vi "writeToXML.vi"(8 "error in (no error)":errorcluster, 10 "Class Label":string="GuideTargetPosition", 11 "GuideTargetPosition in":refnum<class "GuideTargetPosition.lvclass">) -> (0 "error out":errorcluster, 2 "outputXMLString":string="<GuideTargetPosition>\n  <target>\n    <gTargTime>0</gTargTime>\n    <trackID>0</trackID>\n    <xPosition_mm>0</xPosition_mm>\n    <yPosition_mm>0</yPosition_mm>\n  </target>\n</GuideTargetPosition>", 3 "GuideTargetPosition out":refnum<class "GuideTargetPosition.lvclass">)   [LabVIEW 2022 SP3, in "TCSDataDefinitions.lvlib" / "TCSGuiderStatus.lvlib" / "GuideTargetPosition.lvclass"]
uses:
  GuideTargetPosition.lvclass
  GuideTargetPosition.lvclass/GuideTargetPosition.ctl
  TCSGuiderStatus/TCSGuideStatus.lvclass
  GWTargetPositionParameters/GWTargetPositionParameters.lvclass
  <userlib>/Common/XML/XMLGenerator/XMLGenerator.lvclass
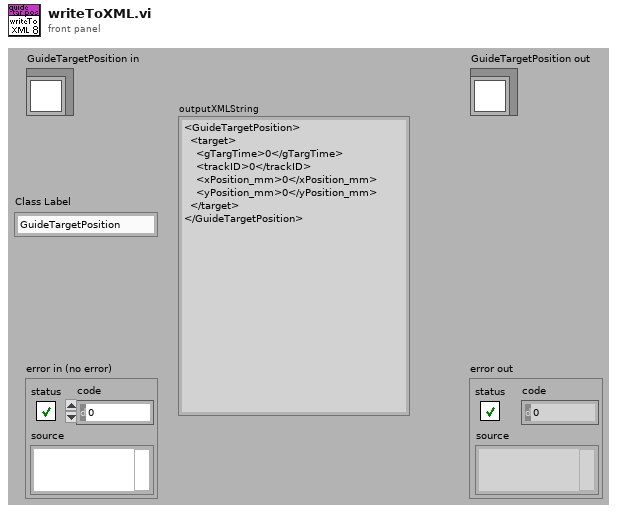
[diagram p1: front panel]
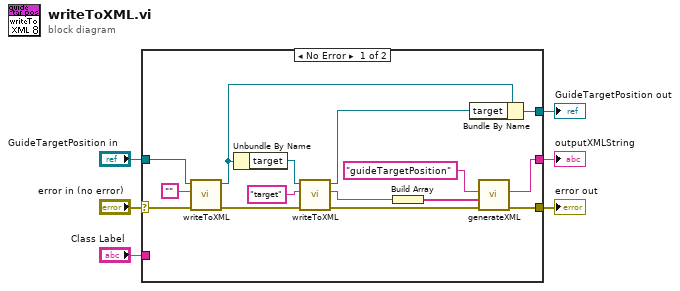
[diagram p0: block diagram]
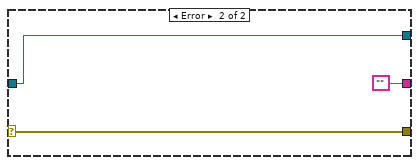
[diagram p2: hidden frame]
diagram:
  n1 = case shown="No Error" "error in (no error)" {
    selector: "error in (no error)" -> [w20 w24]
    tunnel: [w10 w24] -> w5
    tunnel: [w16 w23] -> w3
    tunnel: "GuideTargetPosition in" -> [w21 w23]
    tunnel: [w12 ""] -> w2
    tunnel: "Class Label" -> [_ _]
    frame No Error {
      n2 = call-parent "writeToXML.vi"("error in (no error)"=w20, "Class label"="", "TCSGuiderStatus in"=w21) -> ("error out"=w17:errorcluster, "TCSGuiderStatus out"=w15:refnum<class "GuideTargetPosition.lvclass">)  [unwired: 6 in, 1 out]
      n3 = Unbundle By Name(w15) -> ("target"=w19:refnum<class "GWTargetPositionParameters.lvclass">)
      n4 = call-dynamic "writeToXML.vi"("error in (no error)"=w17, "Class Label"="target", "GWTargetPositionParameters in"=w19) -> ("error out"=w11:errorcluster, "outputXMLString"=w13:string, "GWTargetPositionParameters out"=w18:refnum<class "GWTargetPositionParameters.lvclass">)  [unwired: 6 in]
      n5 = Build Array(w13) -> (w14:string[])
      n6 = Bundle By Name(cluster=w15, "target"=w18) -> (w16:refnum<class "GuideTargetPosition.lvclass">)
      n7 = call <userlib>:"generateXML.vi"("error in"=w11, "childrenXML"=w14, "elementName"="guideTargetPosition" ("Class Label")) -> ("error out"=w10:errorcluster, "XML out"=w12:string)  [unwired: 6 in, 1 out]
    }
    frame Error {
    }
  }
  "error out" <- w5
  "GuideTargetPosition out" <- w3
  "outputXMLString" <- w2
